vi "Bottle_test_status_string.vi"(6 "curent bottle":i32, 7 "i of bottles":i32, 9 "n of repetitions":i32, 10 "i repetition":i32, 11 "n of bottles":i32) -> (3 "Status":string)   [LabVIEW 2016]
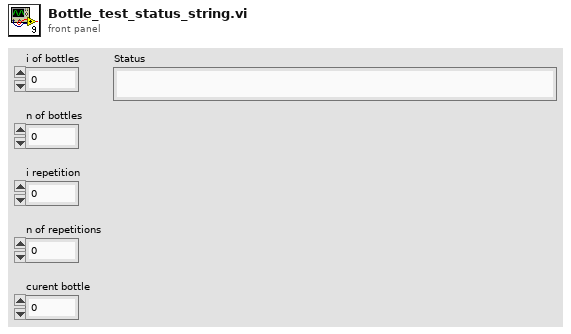
[diagram p1: front panel]
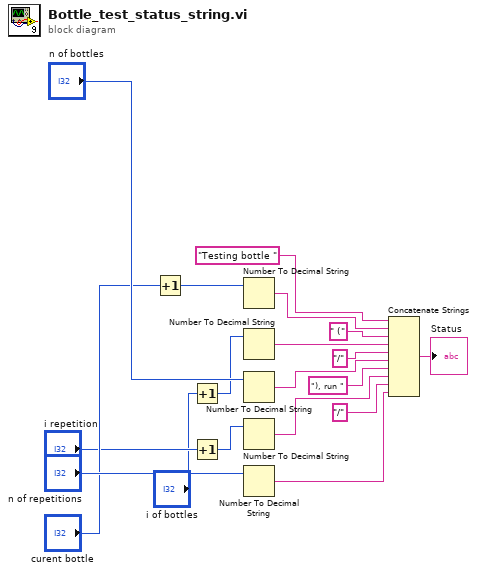
[diagram p0: block diagram]
diagram:
  n1 = Increment(x="curent bottle") -> (x+1=w19:i32)
  n2 = Increment(x="i of bottles") -> (x+1=w7:i32)
  n3 = Increment(x="i repetition") -> (x+1=w10:i32)
  n4 = Number To Decimal String(number=w19) -> (decimal integer string=w2:string)  [unwired: 1 in]
  n5 = Number To Decimal String(number=w7) -> (decimal integer string=w5:string)  [unwired: 1 in]
  n6 = Number To Decimal String(number="n of bottles") -> (decimal integer string=w8:string)  [unwired: 1 in]
  n7 = Number To Decimal String(number=w10) -> (decimal integer string=w12:string)  [unwired: 1 in]
  n8 = Number To Decimal String(number="n of repetitions") -> (decimal integer string=w14:string)  [unwired: 1 in]
  n9 = Concatenate Strings("Testing bottle " ("string"), w2, " (" ("string"), w5, "/" ("string"), w8, "), run " ("string"), w12, "/" ("string"), w14) -> (→"Status":string)
